vi "Get All Data Channels.vi"(8 "error in (no error)":errorcluster, 11 "Framework Ref in":T1 format="%.0x") -> (0 "error out":errorcluster, 2 "Channels refs":T1[](array[typedef]) format="%.0x", 3 "Framework Ref out":T1 format="%.0x")   [LabVIEW 2017, in "DSF Shared.lvlib"]
uses:
  DSF Shared.lvlib
  <vilib>/NI Veristand/Custom Device API/Custom Device Item Ref.ctl
  <vilib>/NI Veristand/Custom Device API/Custom Device API.lvlib
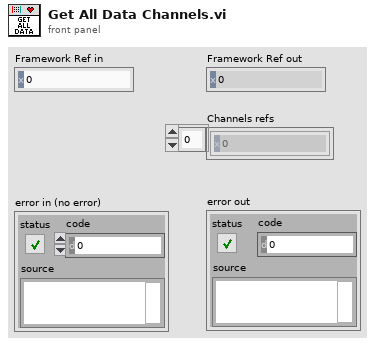
[diagram p1: front panel]
types:
  T1 = typedef "Custom Device API.lvlib/Custom Device Item Ref.ctl" = u64
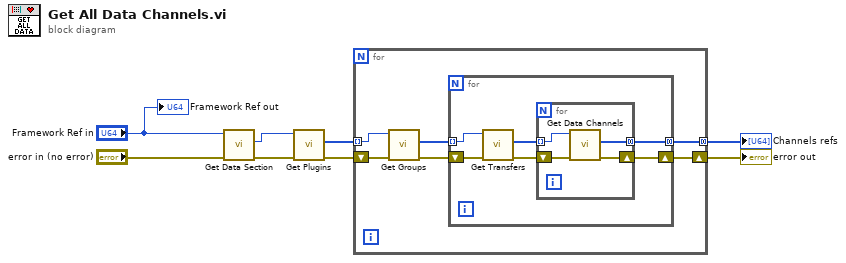
[diagram p0: block diagram]
diagram:
  n1 = call "Get Data Section.vi"("error in (no error)"="error in (no error)", "Item Ref in"="Framework Ref in") -> ("error out"=w4:errorcluster, "Data Section ref"=w3:T1)  [unwired: 6 in, 2 out]
  n2 = call "Get Plugins.vi"("error in (no error)"=w4, "Item Ref in"=w3) -> ("error out"=w8:errorcluster, "Plugin refs"=w7:T1[])  [unwired: 7 in, 1 out]
  n3 = for {
    shift-right: [w10] -> w2
    shift-left: w8 -> [w14]
    tunnel: w7 -> [w13] mode=indexing
    tunnel: [w9] -> w1 mode=concatenating
    n4 = call "Get Groups.vi"("error in (no error)"=w14, "Plugin Ref in"=w13) -> ("error out"=w12:errorcluster, "Group refs"=w11:T1[])  [unwired: 7 in, 1 out]
    n5 = for {
      shift-right: [w15] -> w10
      shift-left: w12 -> [w20]
      tunnel: w11 -> [w19] mode=indexing
      tunnel: [w16] -> w9 mode=concatenating
      n6 = call "Get Transfers.vi"("error in (no error)"=w20, "Group Ref in"=w19) -> ("error out"=w18:errorcluster, "Transfer refs"=w17:T1[])  [unwired: 7 in, 1 out]
      n7 = for {
        shift-right: [w22] -> w15
        shift-left: w18 -> [w24]
        tunnel: w17 -> [w23] mode=indexing
        tunnel: [w21] -> w16 mode=concatenating
        n8 = call "Get Data Channels.vi"("error in (no error)"=w24, "Transfer Ref in"=w23) -> ("error out"=w22:errorcluster, "Channels refs"=w21:T1[])  [unwired: 7 in, 1 out]
      }
    }
  }
  "error out" <- w2
  "Channels refs" <- w1
  "Framework Ref out" <- "Framework Ref in"
